vi "checkVisa.vi"(8 "error in (no error)":errorcluster, 11 "SR430Class in":refnum<class "SR430Class.lvclass">) -> (0 "error out":errorcluster, 3 "SR430Class out":refnum<class "SR430Class.lvclass">)   [LabVIEW 2015, in "SR430Class.lvclass"]
uses:
  class/SR430Class.lvclass
  class/SR430Class.lvclass/SR430Class.ctl
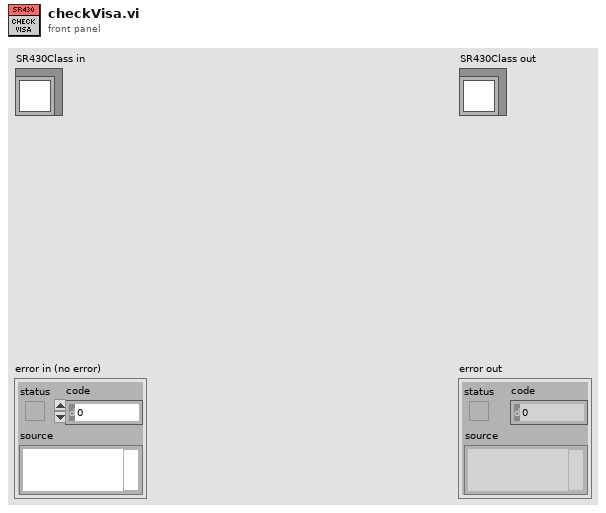
[diagram p1: front panel]
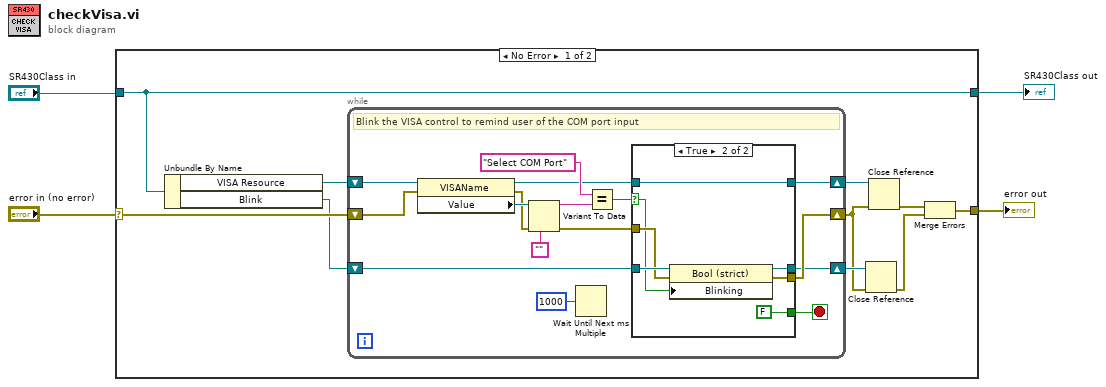
[diagram p0: block diagram]
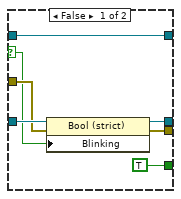
[diagram p2: hidden frame]
diagram:
  n1 = case shown="No Error" "error in (no error)" {
    selector: "error in (no error)" -> [w12 w46]
    tunnel: [w8 w46] -> w3
    tunnel: [w11 w45] -> w1
    tunnel: "SR430Class in" -> [w11 w45]
    frame No Error {
      n2 = Unbundle By Name(w11) -> ("VISA Resource"=w14:refnum<vi>, "Blink"=w10:refnum<vi>)
      n3 = while {
        shift-right: [w23] -> w13
        shift-left: w14 -> [w17]
        shift-right: [w22] -> w6
        shift-left: w12 -> [w21]
        shift-right: [w15] -> w7
        shift-left: w10 -> [w16]
        stop <- w19 stop-if-true
        # "Blink the VISA control to remind user of the COM port input"
        n4 = property class="VISAName"(reference=w17, error in=w21) -> (reference out=w25:refnum<vi>, error out=w28:errorcluster, "Value"=w29:refnum<visa-resource-name>)
        n5 = Variant To Data(error in=w28, type="", Variant=w29) -> (data=w26:string, error out=w20:errorcluster)
        n6 = Wait Until Next ms Multiple(millisecond multiple=u32 1000) -> ()  [unwired: 1 out]
        n7 = Equal?(x="Select COM Port" ("y"), y=w26) -> (x = y?=w24:bool)
        n8 = case shown="True" w24 {
          selector: w24 -> [w31 w39]
          tunnel: w25 -> [w37 w40]
          tunnel: [w37 w40] -> w23
          tunnel: [w32 w41] -> w22
          tunnel: w20 -> [w33 w42]
          tunnel: [TRUE FALSE] -> w19
          tunnel: w16 -> [w35 w43]
          tunnel: [w34 w38] -> w15
          frame False {
            n9 = property class="Bool (strict)"(reference=w35, error in=w33, "Blinking"=w31) -> (reference out=w34:refnum<vi>, error out=w32:errorcluster)
          }
          frame True {
            n10 = property class="Bool (strict)"(reference=w43, error in=w42, "Blinking"=w39) -> (reference out=w38:refnum<vi>, error out=w41:errorcluster)
          }
        }
      }
      n11 = Close Reference(reference=w7, error in (no error)=w6) -> (error out=w5:errorcluster)
      n12 = Close Reference(reference=w13, error in (no error)=w6) -> (error out=w9:errorcluster)
      n13 = Merge Errors(w9, w5) -> (w8:errorcluster)
    }
    frame Error {
    }
  }
  "error out" <- w3
  "SR430Class out" <- w1
